vi "Ping API.vi"(8 "Error in":errorcluster caption="Error in (no error)") -> (0 "Error out":errorcluster, 3 "Connection OK":bool)   [LabVIEW 2018]
uses:
  <vilib>/httpClient/LabVIEWHTTPClient.lvlib
  <vilib>/GPower/Error/GPError.lvlib
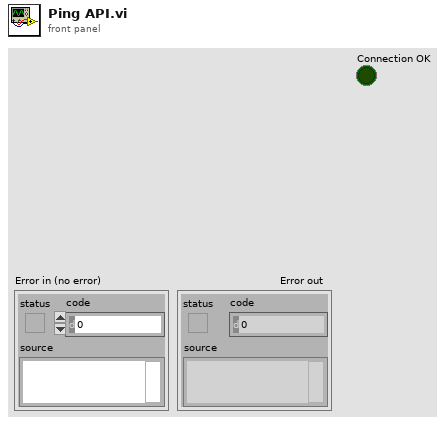
[diagram p1: front panel]
types:
  T1 = typedef "LabVIEWHTTPClient.lvlib/ClientHandle.ctl" = refnum<k1>
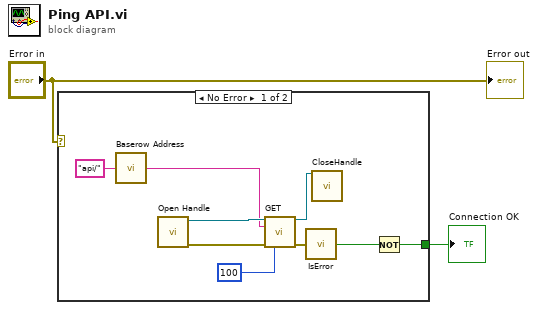
[diagram p0: block diagram]
diagram:
  n1 = case shown="No Error" "Error in" {
    tunnel: [w5 _] -> w1
    frame No Error {
      n2 = call "Baserow Address.vi"("Path"="api/" ("url")) -> ("URL + Path"=w3:string)
      n3 = call "Open Handle.vi"() -> ("error out"=w11:errorcluster, "Refnum out"=w9:T1)  [unwired: 10 in]
      n4 = call <vilib>:"GET.vi"("client handle"=w9, "url"=w3, "error in (no error)"=w11, "timeout (10000)"=100) -> ("client handle out"=w10:T1, "error out"=w7:errorcluster)  [unwired: 8 in, 2 out]
      n5 = call <vilib>:"IsError.vi"("Error in"=w7) -> ("Error?"=w6:bool)  [unwired: 4 in]
      n6 = call <vilib>:"CloseHandle.vi"("client handle"=w10) -> ()  [unwired: 14 in, 1 out]
      n7 = Not(x=w6) -> (.not. x?=w5:bool)
    }
    frame Error {
    }
  }
  "Connection OK" <- w1
  "Error out" <- "Error in"
